vi "CloseEverything.vi"() -> (0 "error out":errorcluster)   [LabVIEW 2010]
uses:
  <userlib>/ROSforLV_0.1/ROS/Code/_ROSDefinition.vi
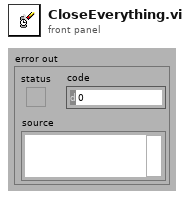
[diagram p1: front panel]
types:
  T1 = cluster{"server vi":string, "reference":refnum<vi>, "Description":string[]}[]
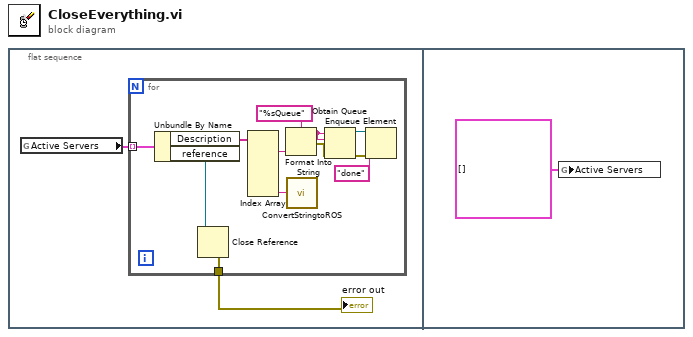
[diagram p0: block diagram]
diagram:
  n1 = flat-sequence {
    frame #0 {
      n2 = global read "_ROSDefinition.vi" "Active Servers"() -> (w1:T1)
      n3 = for {
        tunnel: [w14] -> w2
        tunnel: w1 -> [w13] mode=indexing
        n4 = Unbundle By Name(w13) -> ("Description"=w5:string[], "reference"=w12:refnum<vi>)
        n5 = Close Reference(reference=w12) -> (error out=w14:errorcluster)  [unwired: 1 in]
        n6 = Index Array(array=w5) -> (element #1=w10:string, element #6=w3:string)  [unwired: 6 in, 4 out]
        n7 = Format Into String(format string="%sQueue" ("name (unnamed)"), w10) -> (resulting string=w8:string, error out=w9:errorcluster)  [unwired: 2 in]
        n8 = call <userlib>:"ConvertStringtoROS.vi"("string in"=w3) -> ()  [unwired: 1 out]
        n9 = Obtain Queue(name (unnamed)=w8, element data type=w8, error in (no error)=w9) -> (queue out=w7:refnum<queue>, error out=w4:errorcluster)  [unwired: 2 in, 1 out]
        n10 = Enqueue Element(queue=w7, element="done", error in (no error)=w4) -> ()  [unwired: 1 in, 3 out]
      }
      "error out" <- w2
    }
    frame #1 {
      n11 = global write "_ROSDefinition.vi" "Active Servers"(T1 [] ("Active Topics")) -> ()
    }
  }
